vi "Write Data Raw reference.vi"(8 "error in (no error)":errorcluster, 11 "Experiment in":refnum<class "Experiment.lvclass">) -> (0 "error out":errorcluster, 3 "Experiment out":refnum<class "Experiment.lvclass">)   [LabVIEW 2015, in "Experiment.lvclass"]
uses:
  Experiment.lvclass
  Experiment.lvclass/Experiment.ctl
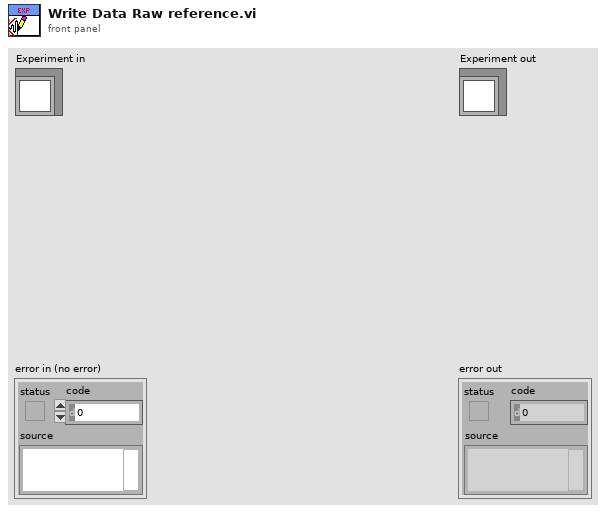
[diagram p1: front panel]
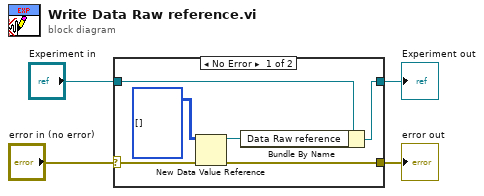
[diagram p0: block diagram]
diagram:
  n1 = case shown="No Error" "error in (no error)" {
    selector: "error in (no error)" -> [w7 w11]
    tunnel: [w5 w11] -> w3
    tunnel: [w9 w12] -> w1
    tunnel: "Experiment in" -> [w10 w12]
    frame No Error {
      n2 = New Data Value Reference(data value=i32[][][][] [], error in=w7) -> (data value reference=w6:refnum<data-value>, error out=w5:errorcluster)
      n3 = Bundle By Name(cluster=w10, "Data Raw reference"=w6) -> (w9:refnum<class "Experiment.lvclass">)
    }
    frame Error {
    }
  }
  "error out" <- w3
  "Experiment out" <- w1
